vi "Simulation-05.vi"() -> (0 "error out":errorcluster, 3 "success":bool)   [LabVIEW 2020]
uses:
  librarian_class/typedefs/book_state--enum.ctl
  shared/request--enum.ctl
  librarian_class/librarian.lvclass
  client_class/client.lvclass
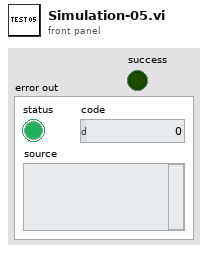
[diagram p1: front panel]
types:
  T1 = typedef "request--enum.ctl" = enum16{"CHECKIN", "CHECKOUT"}
  T2 = typedef "librarian.lvclass/book_state--enum.ctl" = enum16{"CHECKEDIN", "CHECKEDOUT", "DAMAGED"}
  T3 = typedef "message--cluster.ctl" = cluster{"header":string, "cmd":T1, "title":string, "book":string}
  T4 = typedef "librarian.lvclass/lib_map_value--cluster.ctl" = cluster{"book state":T2, "text":string, "hash":string}
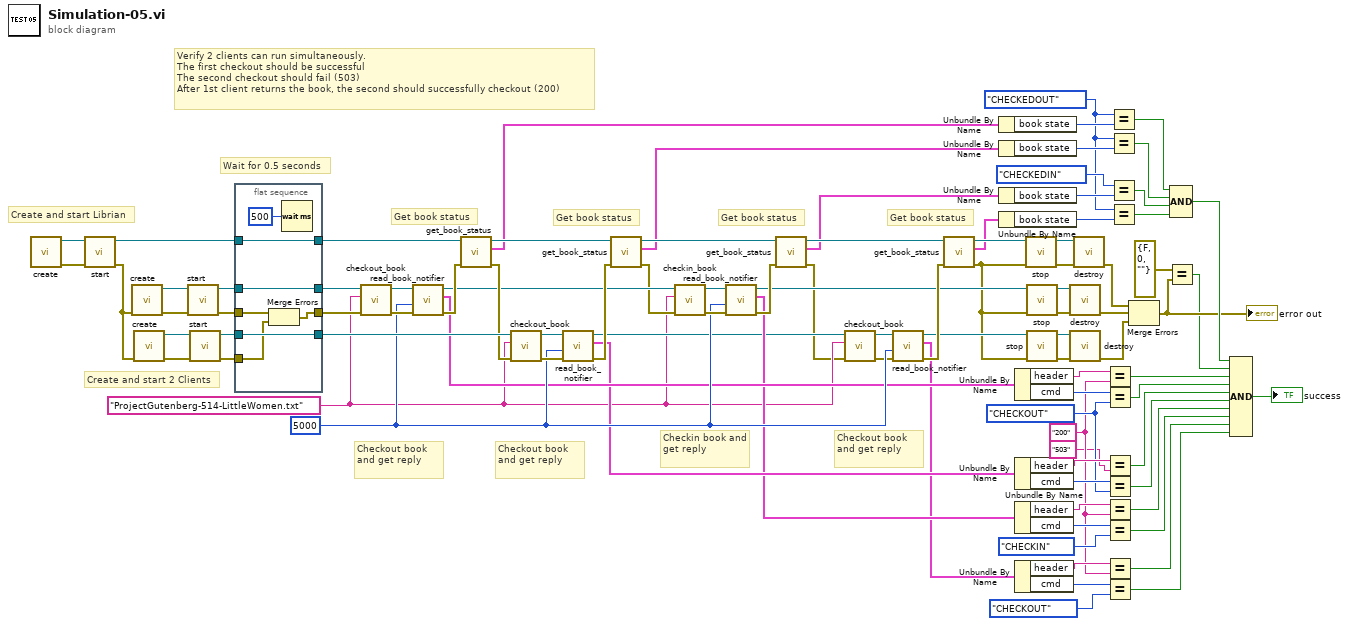
[diagram p0: block diagram]
diagram:
  w33 = request--enum."CHECKOUT" ("y")
  w27 = "200" ("x")
  w1 = book_state--enum."CHECKEDOUT" ("x")
  w65 = 5000 ("timeout in ms (-1)")
  w6 = "ProjectGutenberg-514-LittleWomen.txt" ("book title")
  # "Verify 2 clients can run simultaneously.  \nThe first checkout should be successful\nThe second checkout should fail (503)\nAfter 1st client returns the book, the second should successfully checkout (200)"
  # "Get book status"
  # "Get book status"
  # "Get book status"
  # "Get book status"
  # "Checkout book and get reply"
  # "Checkin book and get reply"
  # "Checkout book and get reply"
  # "Checkout book and get reply"
  # "Wait for 0.5 seconds"
  # "Create and start 2 Clients"
  # "Create and start Librian"
  n1 = call "create.vi"() -> ("error out"=w94:errorcluster, "librarian_sm out"=w95:refnum<class "librarian.lvclass">)  [unwired: 10 in]
  n2 = call "start.vi"("error in (no error)"=w94, "librarian_sm in"=w95) -> ("error out"=w90:errorcluster, "librarian_sm out"=w89:refnum<class "librarian.lvclass">)  [unwired: 8 in]
  n3 = call "create.vi"("error in (no error)"=w90) -> ("error out"=w92:errorcluster, "librarian_sm out"=w93:refnum<class "client.lvclass">)  [unwired: 9 in]
  n4 = call "create.vi"("error in (no error)"=w90) -> ("error out"=w86:errorcluster, "librarian_sm out"=w91:refnum<class "client.lvclass">)  [unwired: 9 in]
  n5 = call "start.vi"("error in (no error)"=w92, "librarian_sm in"=w93) -> ("error out"=w88:errorcluster, "librarian_sm out"=w85:refnum<class "client.lvclass">)  [unwired: 8 in]
  n6 = call "start.vi"("error in (no error)"=w86, "librarian_sm in"=w91) -> ("error out"=w87:errorcluster, "librarian_sm out"=w84:refnum<class "client.lvclass">)  [unwired: 8 in]
  n7 = flat-sequence {
    tunnel: w89 -> [w102]
    tunnel: w88 -> [w98]
    tunnel: w87 -> [w97]
    tunnel: w85 -> [w101]
    tunnel: w84 -> [w100]
    tunnel: [w102] -> w76
    tunnel: [w101] -> w82
    tunnel: [w96] -> w81
    tunnel: [w100] -> w77
    frame #0 {
      n8 = Merge Errors(w98, w97) -> (w96:errorcluster)
      n9 = Wait (ms)(milliseconds to wait=u32 500) -> ()  [unwired: 1 out]
    }
  }
  n10 = call "checkout_book.vi"("error in (no error)"=w81, "book title"=w6, "client in"=w82) -> ("error out"=w80:errorcluster, "client out"=w83:refnum<class "client.lvclass">)  [unwired: 7 in]
  n11 = call "read_book_notifier.vi"("error in (no error)"=w80, "timeout in ms (-1)"=w65, "client in"=w83) -> ("error out"=w75:errorcluster, "msg"=w26:T3, "client out"=w71:refnum<class "client.lvclass">)  [unwired: 6 in]
  n12 = call "get_book_status.vi"("error in (no error)"=w75, "librarian in"=w76) -> ("error out"=w74:errorcluster, "book status"=w47:T4, "librarian out"=w73:refnum<class "librarian.lvclass">)  [unwired: 7 in]
  n13 = call "checkout_book.vi"("error in (no error)"=w74, "book title"=w6, "client in"=w77) -> ("error out"=w79:errorcluster, "client out"=w78:refnum<class "client.lvclass">)  [unwired: 7 in]
  n14 = call "read_book_notifier.vi"("error in (no error)"=w79, "timeout in ms (-1)"=w65, "client in"=w78) -> ("error out"=w72:errorcluster, "msg"=w25:T3, "client out"=w7:refnum<class "client.lvclass">)  [unwired: 6 in]
  n15 = call "get_book_status.vi"("error in (no error)"=w72, "librarian in"=w73) -> ("error out"=w70:errorcluster, "book status"=w46:T4, "librarian out"=w66:refnum<class "librarian.lvclass">)  [unwired: 7 in]
  n16 = call "checkin_book.vi"("error in (no error)"=w70, "book title"=w6, "client in"=w71) -> ("error out"=w69:errorcluster, "client out"=w68:refnum<class "client.lvclass">)  [unwired: 7 in]
  n17 = call "read_book_notifier.vi"("error in (no error)"=w69, "timeout in ms (-1)"=w65, "client in"=w68) -> ("error out"=w67:errorcluster, "msg"=w24:T3, "client out"=w59:refnum<class "client.lvclass">)  [unwired: 6 in]
  n18 = call "get_book_status.vi"("error in (no error)"=w67, "librarian in"=w66) -> ("error out"=w5:errorcluster, "book status"=w43:T4, "librarian out"=w64:refnum<class "librarian.lvclass">)  [unwired: 7 in]
  n19 = call "checkout_book.vi"("error in (no error)"=w5, "book title"=w6, "client in"=w7) -> ("error out"=w9:errorcluster, "client out"=w8:refnum<class "client.lvclass">)  [unwired: 7 in]
  n20 = call "read_book_notifier.vi"("error in (no error)"=w9, "timeout in ms (-1)"=w65, "client in"=w8) -> ("error out"=w63:errorcluster, "msg"=w23:T3, "client out"=w61:refnum<class "client.lvclass">)  [unwired: 6 in]
  n21 = call "get_book_status.vi"("error in (no error)"=w63, "librarian in"=w64) -> ("error out"=w52:errorcluster, "book status"=w42:T4, "librarian out"=w53:refnum<class "librarian.lvclass">)  [unwired: 7 in]
  n22 = Unbundle By Name(w47) -> ("book state"=w49:T2)
  n23 = Unbundle By Name(w46) -> ("book state"=w48:T2)
  n24 = Unbundle By Name(w43) -> ("book state"=w44:T2)
  n25 = Unbundle By Name(w42) -> ("book state"=w45:T2)
  n26 = Unbundle By Name(w26) -> ("header"=w36:string, "cmd"=w37:T1)
  n27 = Unbundle By Name(w25) -> ("header"=w34:string, "cmd"=w35:T1)
  n28 = Unbundle By Name(w24) -> ("header"=w29:string, "cmd"=w28:T1)
  n29 = Unbundle By Name(w23) -> ("header"=w31:string, "cmd"=w30:T1)
  n30 = call "stop.vi"("error in (no error)"=w52, "librarian_sm in"=w53) -> ("error out"=w50:errorcluster, "librarian_sm out"=w54:refnum<class "librarian.lvclass">)  [unwired: 8 in]
  n31 = call "stop.vi"("error in (no error)"=w52, "librarian_sm in"=w59) -> ("error out"=w58:errorcluster, "librarian_sm out"=w60:refnum<class "client.lvclass">)  [unwired: 8 in]
  n32 = call "stop.vi"("error in (no error)"=w52, "librarian_sm in"=w61) -> ("error out"=w57:errorcluster, "librarian_sm out"=w62:refnum<class "client.lvclass">)  [unwired: 8 in]
  n33 = call "destroy.vi"("error in (no error)"=w58, "librarian_sm in"=w60) -> ("error out"=w56:errorcluster)  [unwired: 8 in, 1 out]
  n34 = call "destroy.vi"("error in (no error)"=w57, "librarian_sm in"=w62) -> ("error out"=w55:errorcluster)  [unwired: 8 in, 1 out]
  n35 = call "destroy.vi"("error in (no error)"=w50, "librarian_sm in"=w54) -> ("error out"=w51:errorcluster)  [unwired: 8 in, 1 out]
  n36 = Equal?(x=w36, y=w27) -> (x = y?=w22:bool)
  n37 = Equal?(x=w37, y=w33) -> (x = y?=w21:bool)
  n38 = Equal?(x=w34, y="503" ("x")) -> (x = y?=w20:bool)
  n39 = Equal?(x=w35, y=w33) -> (x = y?=w19:bool)
  n40 = Equal?(x=w29, y=w27) -> (x = y?=w18:bool)
  n41 = Equal?(x=w28, y=request--enum."CHECKIN") -> (x = y?=w17:bool)
  n42 = Equal?(x=w31, y=w27) -> (x = y?=w16:bool)
  n43 = Equal?(x=w30, y=request--enum."CHECKOUT") -> (x = y?=w15:bool)
  n44 = Equal?(x=w1, y=w49) -> (x = y?=w38:bool)
  n45 = Equal?(x=w1, y=w48) -> (x = y?=w39:bool)
  n46 = Equal?(x=book_state--enum."CHECKEDIN", y=w44) -> (x = y?=w40:bool)
  n47 = Equal?(x=w1, y=w45) -> (x = y?=w41:bool)
  n48 = Merge Errors(w51, w56, w55) -> (w12:errorcluster)
  "error out" <- w12
  n49 = Equal?(x=errorcluster {"status"=FALSE, "code"=0, "source"=""} ("y"), y=w12) -> (x = y?=w11:bool)
  n50 = Compound Arithmetic op=AND(w38, w39, w40, w41) -> (w14:bool)
  n51 = Compound Arithmetic op=AND(w14, w11, w22, w21, w20, w19, w18, w17, w16, w15) -> (→"success":bool)
